vi "SIM_Drive_MODULE_EXECUTE.vi"(7 "Module Index":i32, 8 "error in (no error)":errorcluster, 9 "Battery Voltage":dbl, 10 "SpinMotorDmd":dbl, 11 "TravelMotorDmd":dbl) -> (0 "error out":errorcluster, 1 "Abs Current":dbl, 2 "ModulePosition":T1={"Distance"=0.0, "Angle"={"VALUE"=0.0, "COS"=1.0, "SIN"=0.0}, "P"=FALSE} {"Angle"."SIN" format="%13.4f"; "Angle"."COS" format="%13.4f"; "Angle"."VALUE" format="%13.4f"}, 3 "ModuleState":T3={"Speed"=0.0, "Angle"={"VALUE"=0.0, "COS"=1.0, "SIN"=0.0}} {"Angle"."SIN" format="%13.4f"; "Angle"."COS" format="%13.4f"; "Angle"."VALUE" format="%13.4f"})   [LabVIEW 2023]
uses:
  <vilib>/Rock Robotics/WPI/ThirdParty/JAS_Junk/TrajLib/TypeDef/SWERVE_DRIVE_MODULE_STATE.ctl
  <vilib>/Rock Robotics/WPI/ThirdParty/JAS_Junk/TrajLib/TypeDef/ROTATION2D.ctl
  <vilib>/Rock Robotics/WPI/ThirdParty/JAS_Junk/TrajLib/TypeDef/SWERVE_DRIVE_MODULE_POSITION.ctl
  <vilib>/Rock Robotics/WPI/ThirdParty/JAS_Junk/TrajLib/Enum/DCMOTOR_TYPES_ENUM.ctl
  <vilib>/Rock Robotics/WPI/ThirdParty/JAS_Junk/TrajLib/MathUtil_InputModulus.vi
  SIM_Drive_Globals.vi
  <vilib>/Rock Robotics/WPI/ThirdParty/JAS_Junk/TrajLib/Trajectory_Library.lvlib
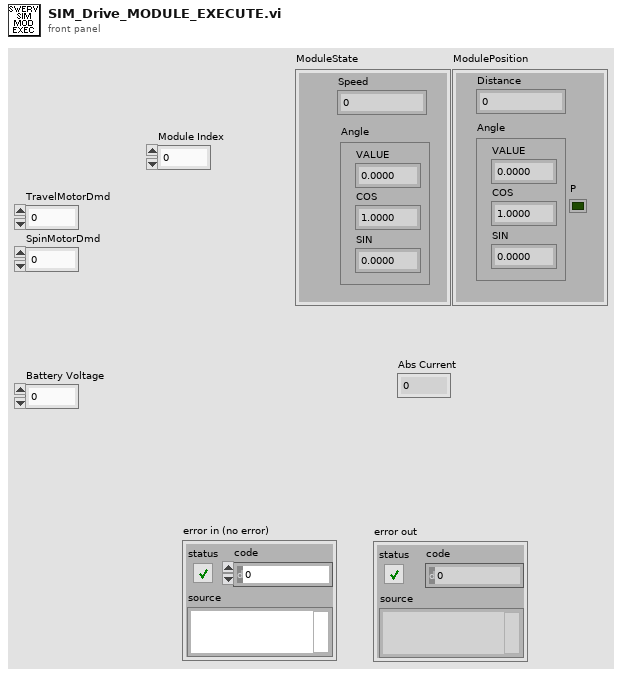
[diagram p1: front panel]
types:
  T1 = typedef "Trajectory_Library.lvlib/SWERVE_DRIVE_MODULE_POSITION.ctl" = cluster{"Distance":dbl, "Angle":T2, "P":bool}
  T2 = typedef "Trajectory_Library.lvlib/ROTATION2D.ctl" = cluster{"VALUE":dbl, "COS":dbl, "SIN":dbl}
  T3 = typedef "Trajectory_Library.lvlib/SWERVE_DRIVE_MODULE_STATE.ctl" = cluster{"Speed":dbl, "Angle":T2}
  T4 = typedef "Trajectory_Library.lvlib/DCMOTOR_TYPES_ENUM.ctl" = enum16{"CIM", "AndyMark 9015", "Andy Mark RS 775 125", "Bag", "BaneBots RS 550", "BaneBots RS 775", "Falcon 500", "Mini CIM", "NEO", "NEO 550", "Romi BuiltIn", "Vex 775 Pro", "Snow Blower AM 2235A", "Bosch Seat AM 3493", "Falcon 500 FOC", "Kraken X60", "Kraken X60 FOC", "NEO Vortex"}
  T5 = cluster{"Swerve Motor Device Index":i32, "Drive Motor Device Index":i32, "Swerve Encoder Device Index":i32, "Drive Encoder Device Index":i32, "Drive DistPerzcount":dbl, "SwerveRadPerCount":dbl}[]
  T6 = typedef "Trajectory_Library.lvlib/LINEAR_SYSTEM_ID_DCMOTOR_MODEL.ctl" = cluster{"DCMOTOR_TYPES":T4, "Num Motors":i32, "Gearing":dbl, "MOI kgm2":dbl}
  T7 = typedef "Trajectory_Library.lvlib/DCMOTOR_SIM_SIMULATION_PARAMS.ctl" = cluster{"Pos Sim Std Dev Rotations":dbl, "Vel Sim Std Dev RPM":dbl}
  T8 = cluster{"Swerve Motor Device Index":i32, "Drive Motor Device Index":i32, "Swerve Encoder Device Index":i32, "Drive Encoder Device Index":i32, "Drive DistPerzcount":dbl, "SwerveRadPerCount":dbl}
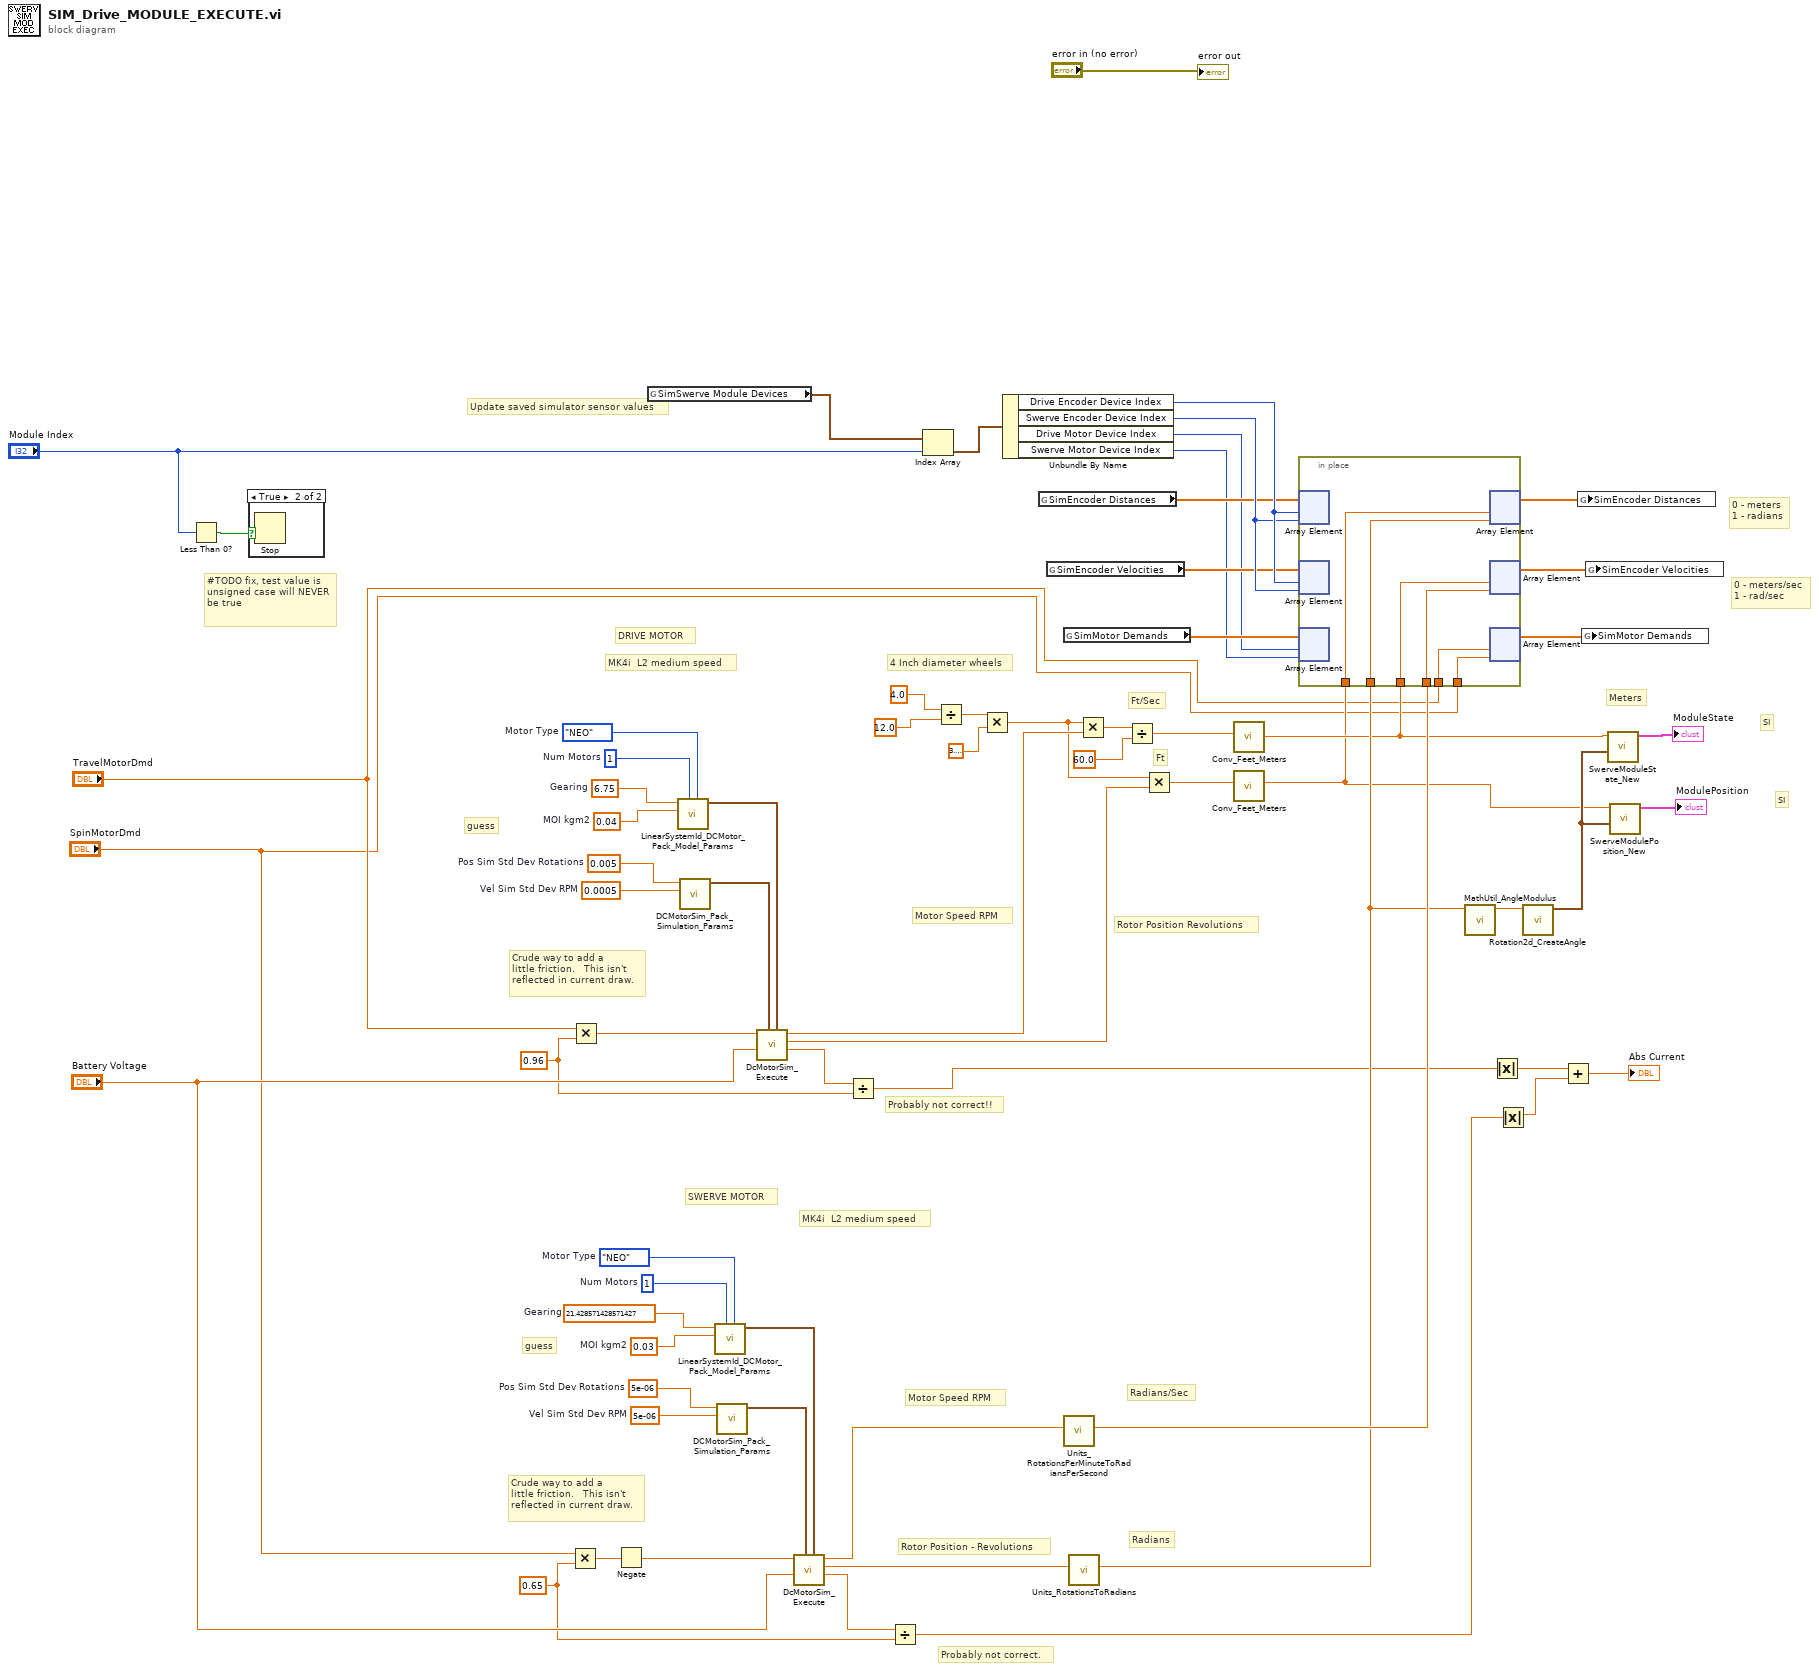
[diagram p0: block diagram]
diagram:
  w13 = 0.96 ("y")
  w11 = 0.65 ("y")
  w41 = 0.005  # Pos Sim Std Dev Rotations
  w42 = 0.0005  # Vel Sim Std Dev RPM
  w45 = 6.75  # Gearing
  w46 = 0.04  # MOI kgm2
  w47 = 1  # Num Motors
  w48 = DCMOTOR_TYPES_ENUM."NEO"  # Motor Type
  w49 = 5e-06  # Pos Sim Std Dev Rotations
  w50 = 5e-06  # Vel Sim Std Dev RPM
  w53 = 21.428571428571427  # Gearing
  w54 = 0.03  # MOI kgm2
  w55 = 1  # Num Motors
  w56 = DCMOTOR_TYPES_ENUM."NEO"  # Motor Type
  # "Probably not correct."
  # "Probably not correct!!"
  # "SI"
  # "SI"
  # "0 - meters \n1 - radians"
  # "0 - meters/sec\n1 - rad/sec"
  # "Crude way to add a \nlittle friction.   This isn't\nreflected in current draw."
  # "Crude way to add a \nlittle friction.   This isn't\nreflected in current draw."
  # "4 Inch diameter wheels"
  # "Radians"
  # "Radians/Sec"
  # "guess"
  # "guess"
  # "Ft/Sec"
  # "Ft"
  # "MK4i  L2 medium speed"
  # "MK4i  L2 medium speed"
  # "Rotor Position Revolutions"
  # "Motor Speed RPM"
  # "Rotor Position - Revolutions"
  # "Motor Speed RPM"
  # "SWERVE MOTOR"
  # "DRIVE MOTOR"
  # "Update saved simulator sensor values"
  # "#TODO fix, test value is unsigned case will NEVER be true"
  # "Meters"
  n1 = Less Than 0?(x="Module Index") -> (x < 0?=w66:bool)
  n2 = case shown="True" w66 {
    frame False {
    }
    frame True {
      n3 = Stop() -> ()  [unwired: 1 in]
    }
  }
  n4 = Multiply(x="SpinMotorDmd", y=w11) -> (x*y=w2:dbl)
  n5 = Multiply(x="TravelMotorDmd", y=w13) -> (x*y=w23:dbl)
  n6 = Negate(x=w2) -> (-x=w1:dbl)
  n7 = global read "SIM_Drive_Globals.vi" "SimSwerve Module Devices"() -> (w65:T5)
  n8 = call <vilib>:"LinearSystemId_DCMotor_Pack_Model_Params.vi"("DCMOTOR_TYPES"=w48, "Num Motors"=w47, "MOI kgm2"=w46, "Gearing"=w45) -> ("LinearSystem_ID_DCMotor_Model"=w44:T6)  [unwired: 7 in]
  n9 = call <vilib>:"DCMotorSim_Pack_Simulation_Params.vi"("Vel Sim Std Dev RPM"=w42, "Pos Sim Std Dev Rotations"=w41) -> ("DCMOTOR_Sim_Simulation_Params"=w43:T7)  [unwired: 9 in]
  n10 = call <vilib>:"LinearSystemId_DCMotor_Pack_Model_Params.vi"("DCMOTOR_TYPES"=w56, "Num Motors"=w55, "MOI kgm2"=w54, "Gearing"=w53) -> ("LinearSystem_ID_DCMotor_Model"=w52:T6)  [unwired: 7 in]
  n11 = call <vilib>:"DCMotorSim_Pack_Simulation_Params.vi"("Vel Sim Std Dev RPM"=w50, "Pos Sim Std Dev Rotations"=w49) -> ("DCMOTOR_Sim_Simulation_Params"=w51:T7)  [unwired: 9 in]
  n12 = call <vilib>:"DcMotorSim_Execute.vi"("DCMotor_Model _Params"=w44, "DCMOTORSim_Simulation_Params"=w43, "Battery Voltage"="Battery Voltage", "Motor Dmd (CO)"=w23) -> ("Motor Current"=w14:dbl, "Position_Rotations"=w34:dbl, "Velocity_RPM"=w36:dbl)  [unwired: 3 in, 2 out]
  n13 = call <vilib>:"DcMotorSim_Execute.vi"("DCMotor_Model _Params"=w52, "DCMOTORSim_Simulation_Params"=w51, "Battery Voltage"="Battery Voltage", "Motor Dmd (CO)"=w1) -> ("Motor Current"=w10:dbl, "Position_Rotations"=w27:dbl, "Velocity_RPM"=w29:dbl)  [unwired: 3 in, 2 out]
  n14 = Divide(x=w14, y=w13) -> (x/y=w12:dbl)
  n15 = Divide(x=w10, y=w11) -> (x/y=w9:dbl)
  n16 = Index Array(array=w65, index="Module Index") -> (element=w64:T8)
  n17 = Divide(x=4.0, y=12.0) -> (x/y=w38:dbl)
  n18 = Multiply(x=w38, y=3.141592653589793) -> (x*y=w35:dbl)
  n19 = Unbundle By Name(w64) -> ("Drive Encoder Device Index"=w63:i32, "Swerve Encoder Device Index"=w62:i32, "Drive Motor Device Index"=w7:i32, "Swerve Motor Device Index"=w6:i32)
  n20 = global read "SIM_Drive_Globals.vi" "SimEncoder Distances"() -> (w61:dbl[])
  n21 = global read "SIM_Drive_Globals.vi" "SimEncoder Velocities"() -> (w60:dbl[])
  n22 = global read "SIM_Drive_Globals.vi" "SimMotor Demands"() -> (w8:dbl[])
  n23 = call <vilib>:"Units_RotationsPerMinuteToRadiansPerSecond.vi"("RotationsPerMinute"=w29) -> ("RadiansPerSecond"=w28:dbl)  [unwired: 10 in]
  n24 = call <vilib>:"Units_RotationsToRadians.vi"("Rotations"=w27) -> ("Radians"=w21:dbl)  [unwired: 10 in]
  n25 = Multiply(x=w35, y=w36) -> (x*y=w33:dbl)
  n26 = Divide(x=w33, y=60.0) -> (x/y=w31:dbl)
  n27 = Multiply(x=w35, y=w34) -> (x*y=w30:dbl)
  n28 = call <vilib>:"Conv_Feet_Meters.vi"("Feet"=w31) -> ("Meters"=w18:dbl)  [unwired: 10 in]
  n29 = call <vilib>:"Conv_Feet_Meters.vi"("Feet"=w30) -> ("Meters"=w17:dbl)  [unwired: 10 in]
  n30 = in-place {
    in-place-border: w21 -> [w70]
    in-place-border: w17 -> [w71]
    in-place-border: w18 -> [w73]
    in-place-border: w28 -> [w72]
    in-place-border: "TravelMotorDmd" -> [w69]
    in-place-border: "SpinMotorDmd" -> [w68]
    n31 = in-place-array #1(w61, w63, w62) -> ()  [unwired: 2 out]
    n32 = in-place-array #2(w60, w63, w62) -> ()  [unwired: 2 out]
    n33 = in-place-array #3(w8, w7, w6) -> ()  [unwired: 2 out]
    n34 = in-place-array #1(w71, w70) -> (w59:dbl[])  [unwired: 2 out]
    n35 = in-place-array #2(w73, w72) -> (w58:dbl[])  [unwired: 2 out]
    n36 = in-place-array #3(w69, w68) -> (w5:dbl[])  [unwired: 2 out]
  }
  n37 = call <vilib>:"MathUtil_AngleModulus.vi"("InputAngle"=w21) -> ("ModulsAngle"=w20:dbl)  [unwired: 10 in]
  n38 = Absolute Value(x=w12) -> (abs(x)=w25:dbl)
  n39 = Absolute Value(x=w9) -> (abs(x)=w24:dbl)
  n40 = call <vilib>:"Rotation2d_CreateAngle.vi"("Angle"=w20) -> ("ROTATION"=w19:T2)  [unwired: 10 in]
  n41 = Add(x=w25, y=w24) -> (x+y=→"Abs Current":dbl)
  n42 = global write "SIM_Drive_Globals.vi" "SimEncoder Distances"(w59) -> ()
  n43 = global write "SIM_Drive_Globals.vi" "SimMotor Demands"(w5) -> ()
  n44 = global write "SIM_Drive_Globals.vi" "SimEncoder Velocities"(w58) -> ()
  n45 = call <vilib>:"SwerveModuleState_New.vi"("ROTATION"=w19, "Speed"=w18) -> ("SWERVE_DRIVE_MODULE_STATE"=→"ModuleState":T3)  [unwired: 9 in]
  n46 = call <vilib>:"SwerveModulePosition_New.vi"("ROTATION"=w19, "Distance"=w17) -> ("SWERVE_DRIVE_MODULE_POSITION"=→"ModulePosition":T1)  [unwired: 9 in]
  "error out" <- "error in (no error)"
